vi "String_Build Name array from Variants.vi"(6 "Array":variant[](array[variant]), 8 "Four":variant, 9 "Three":variant, 10 "Two":variant, 11 "One":variant) -> (3 "Name Array Out":string[](array[string]))   [LabVIEW 2020]
uses:
  <vilib>/Utility/VariantDataType/VariantType.lvlib
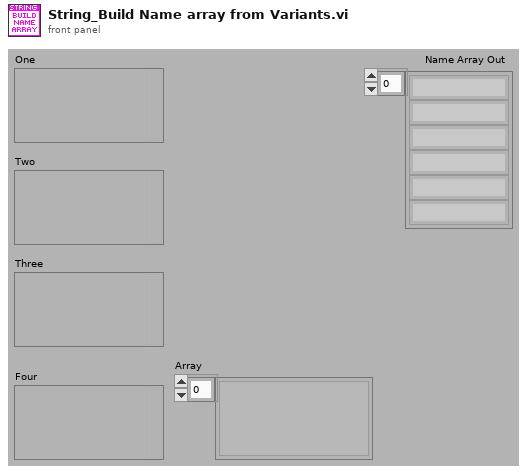
[diagram p1: front panel]
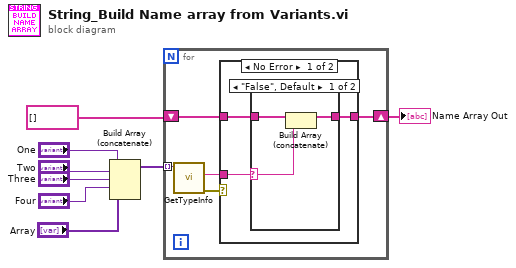
[diagram p0: block diagram]
diagram:
  n1 = Build Array (concatenate)("One", "Two", "Three", "Four", "Array") -> (w8:variant[])
  n2 = for {
    tunnel: w8 -> [w13] mode=indexing
    shift-right: [w9] -> w1
    shift-left: string[] [] ("Name array") -> [w10]
    n3 = call <vilib>:"GetTypeInfo.vi"("Variant"=w13) -> ("error out"=w12:errorcluster, "Name"=w11:string)  [unwired: 6 in, 3 out]
    n4 = case shown="No Error" w12 {
      tunnel: w11 -> [w16 _]
      tunnel: w10 -> [w15 w21]
      tunnel: [w14 w21] -> w9
      frame No Error {
        n5 = case shown="\"False\", Default" w16 {
          selector: w16 -> [w17 _]
          tunnel: w15 -> [w19 w20]
          tunnel: [w18 w20] -> w14
          frame "False", Default {
            n6 = Build Array (concatenate)(w19, w17) -> (w18:string[])
          }
          frame "" {
          }
        }
      }
      frame Error {
      }
    }
  }
  "Name Array Out" <- w1
